vi "Close.vi"(8 "error in (no error)":errorcluster, 11 "Keysight 6700C in":refnum<class "Keysight 6700C.lvclass">) -> (0 "error out":errorcluster, 3 "Keysight 6700C out":refnum<class "Keysight 6700C.lvclass">)   [LabVIEW 2025, in "Power Supply.lvlib" / "Keysight 6700C.lvclass"]
uses:
  Keysight 6700C.lvclass
  Keysight 6700C.lvclass/Keysight 6700C.ctl
  <instrlib>/Agilent N6700 Series/Agilent N6700 Series.lvlib
  PS Instrument/Power Supply Instrument.lvclass
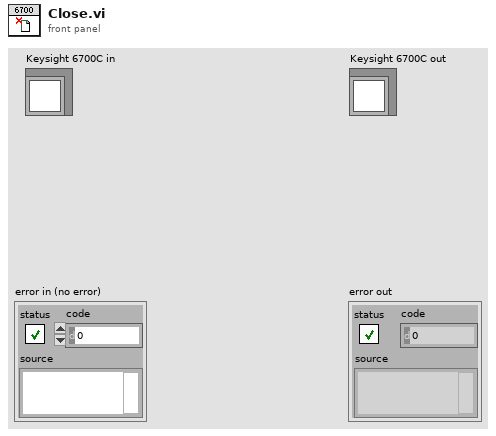
[diagram p1: front panel]
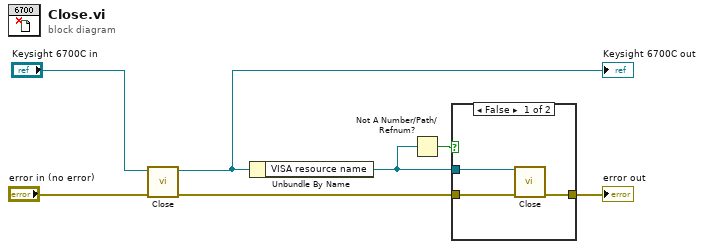
[diagram p0: block diagram]
diagram:
  n1 = call-parent <instrlib>:"Close.vi"("error in (no error)"="error in (no error)", "Power Supply Instrument in"="Keysight 6700C in") -> ("error out"=w3:errorcluster, "Power Supply Instrument out"=w1:refnum<class "Keysight 6700C.lvclass">)  [unwired: 8 in]
  "Keysight 6700C out" <- w1
  n2 = Unbundle By Name(w1) -> ("VISA resource name"=w5:refnum<visa-resource-name>)
  n3 = Not A Number/Path/Refnum?(number/path/refnum=w5) -> (NaN/Path/Refnum?=w4:bool)
  n4 = case shown="False" w4 {
    tunnel: w3 -> [w10 w11]
    tunnel: [w9 w11] -> w6
    tunnel: w5 -> [w8 _]
    frame False {
      n5 = call <instrlib>:"Close.vi"("VISA resource name"=w8, "error in (no error)"=w10) -> ("error out"=w9:errorcluster)  [unwired: 13 in]
    }
    frame True {
    }
  }
  "error out" <- w6
